vi "error_handler_display_loops.vi"(8 "error in (no error)":errorcluster, 11 "Name of VI or Module":string) -> (0 "error out":errorcluster)   [LabVIEW 2020, in "main.lvlib"]
doc: "Blank VI with error handling."
uses:
  main.lvlib
  status_text_indicator/Status_Text_Indicator.lvlib
panel:
  # "Development\ncontrols/indicators useful for development and testing, but which are not outputs of the VI"
  # "Input\nInputs to the VI"
  # "Output\nOutputs of the VI"
  # "Description\n\nBlank VI with error handling case. \n\nSummarize the use of this VI in this space."
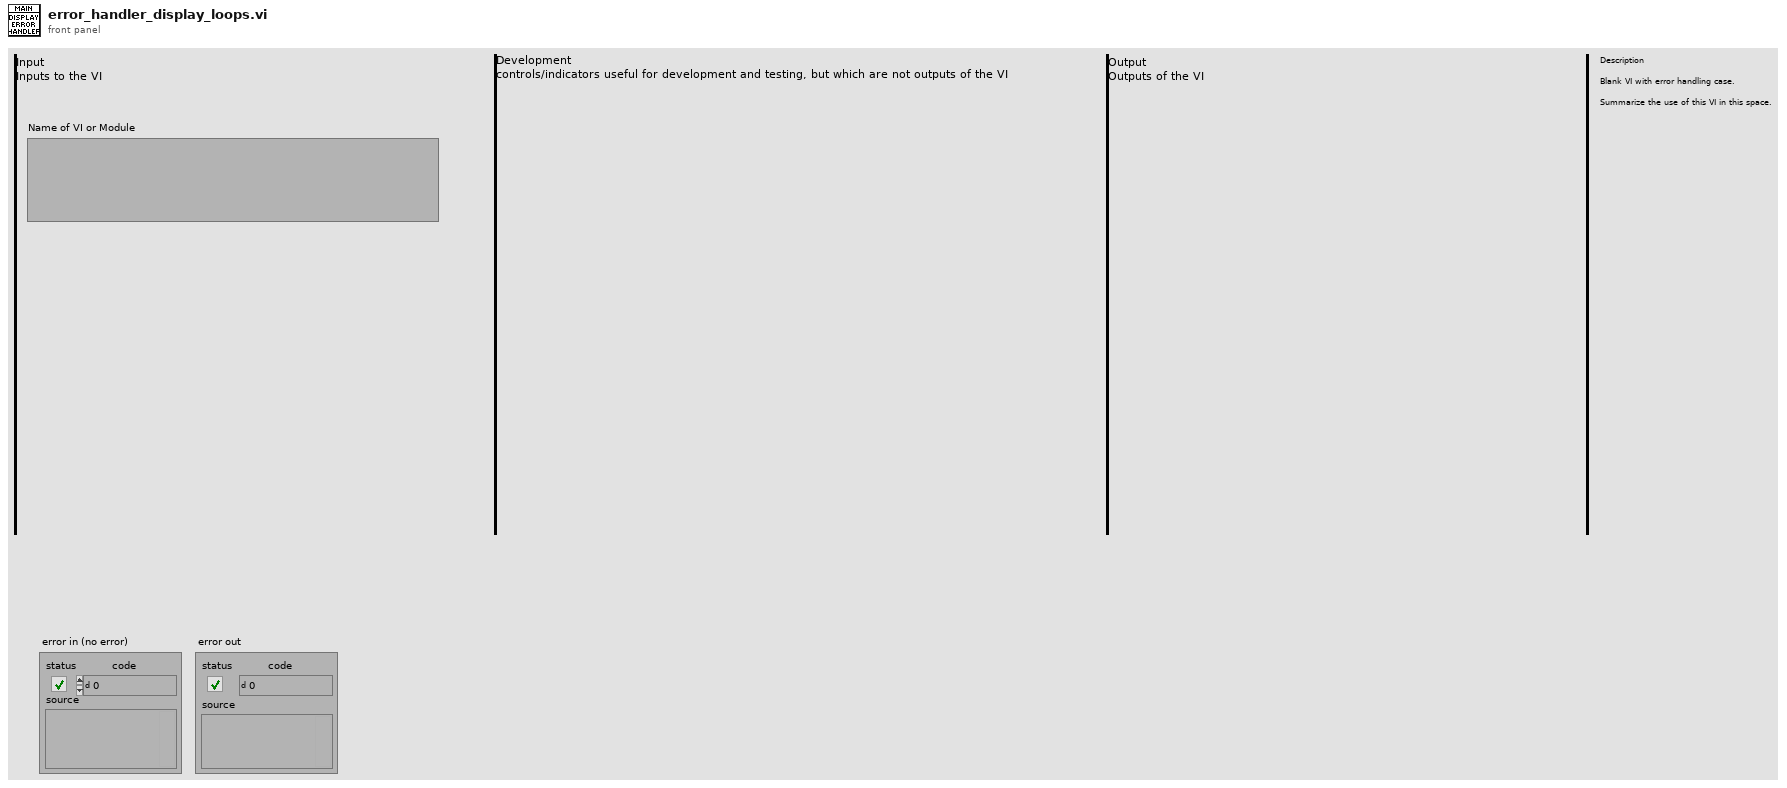
[diagram p1: front panel]
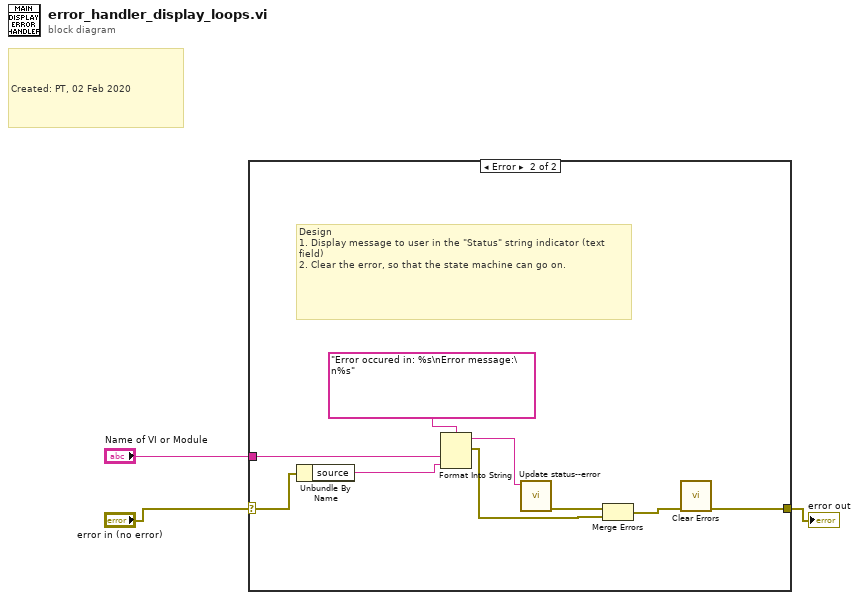
[diagram p0: block diagram]
diagram:
  # "Created: PT, 02 Feb 2020"
  n1 = case shown="Error" "error in (no error)" {
    selector: "error in (no error)" -> [w4 w12]
    tunnel: [w4 w9] -> w2
    tunnel: "Name of VI or Module" -> [_ w5]
    frame No Error {
      # "No error. Good. Nothing to do."
    }
    frame Error {
      # "Design\n1. Display message to user in the \"Status\" string indicator (text field)\n2. Clear the error, so that the state machine can go on."
      n2 = Unbundle By Name(w12) -> ("source"=w6:string)
      n3 = Format Into String(format string="Error occured in: %s\nError message:\n%s", w5, w6) -> (resulting string=w11:string, error out=w7:errorcluster)  [unwired: 2 in]
      n4 = call "Update status--error.vi"("Error message"=w11) -> ("error out"=w10:errorcluster)  [unwired: 10 in]
      n5 = Merge Errors(w10, w7) -> (w8:errorcluster)
      n6 = call <vilib>:"Clear Errors.vi"("error in (no error)"=w8) -> ("error out"=w9:errorcluster)  [unwired: 5 in, 1 out]
    }
  }
  "error out" <- w2
